vi "RTM - Remove Packet.vi"(8 "error in (no error)":errorcluster, 11 "Node Ptr":T1 format="%.0x") -> (0 "error out":errorcluster)   [LabVIEW 2019, in "UDP-Custom-Device System Explorer.lvlib"]
uses:
  UDP-Custom-Device System Explorer.lvlib
  <vilib>/NI VeriStand/Custom Device API/Custom Device Item Ref.ctl
  <vilib>/NI VeriStand/Custom Device Tools/Custom Device Utility Library/Custom Device Utility Library.lvlib
  <vilib>/NI VeriStand/Custom Device API/Custom Device API.lvlib
  Property Accessors/Shared Section Accessors.lvlib
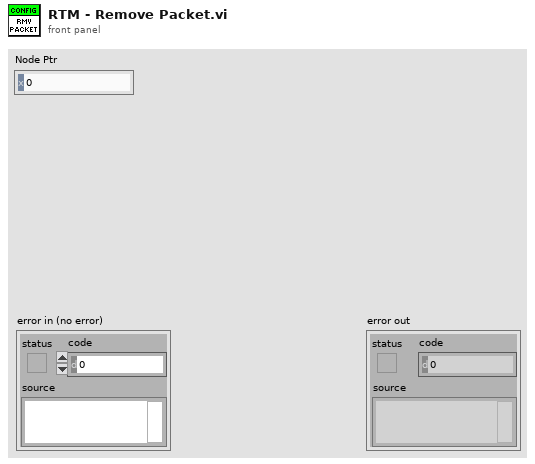
[diagram p1: front panel]
types:
  T1 = typedef "Custom Device API.lvlib/Custom Device Item Ref.ctl" = u64
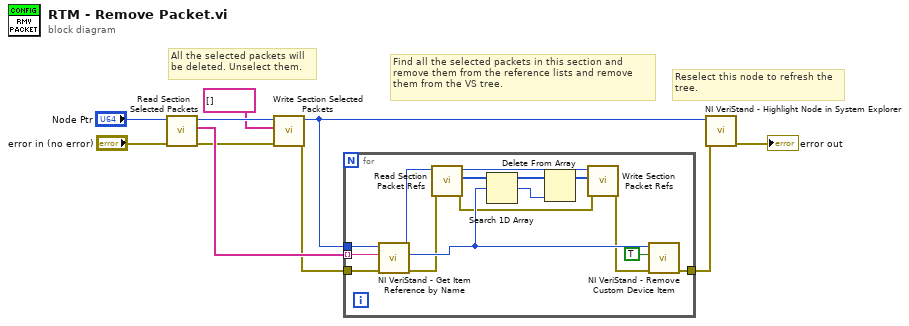
[diagram p0: block diagram]
diagram:
  # "All the selected packets will\nbe deleted. Unselect them."
  # "Reselect this node to refresh the\ntree."
  # "Find all the selected packets in this section and\nremove them from the reference lists and remove\nthem from the VS tree."
  n1 = call "Read Section Selected Packets.vi"("error in (no error)"="error in (no error)", "Node Ptr"="Node Ptr") -> ("error out"=w5:errorcluster, "Selected Packets"=w8:string[], "Node Ptr out"=w7:T1)  [unwired: 7 in]
  n2 = call "Write Section Selected Packets.vi"("error in (no error)"=w5, "Selected Packets"=string[] [] ("Value"), "Node Ptr"=w7) -> ("error out"=w4:errorcluster, "Node Ptr out"=w6:T1)  [unwired: 7 in]
  n3 = for {
    tunnel: w8 -> [w21] mode=indexing
    tunnel: w4 -> [w20]
    tunnel: [w24] -> w10
    tunnel: w6 -> [w22]
    n4 = call <vilib>:"NI VeriStand - Get Item Reference by Name.vi"("error in (no error)"=w20, "Item Name"=w21, "Parent Ref in"=w22) -> ("error out"=w13:errorcluster, "Item Ref"=w18:T1, "Parent Ref out"=w16:T1)  [unwired: 5 in, 1 out]
    n5 = call "Read Section Packet Refs.vi"("error in (no error)"=w13, "Node Ptr"=w16) -> ("error out"=w11:errorcluster, "Dependent Node Refs"=w15:T1[], "Node Ptr out"=w17:T1)  [unwired: 7 in]
    n6 = Search 1D Array(1D array=w15, element=w18) -> (index of element=w19:i32)  [unwired: 1 in]
    n7 = Delete From Array(array=w15, index=w19) -> (array with subset deleted=w14:T1[])  [unwired: 1 in, 1 out]
    n8 = call "Write Section Packet Refs.vi"("error in (no error)"=w11, "Dependent Node Refs"=w14, "Node Ptr"=w17) -> ("error out"=w12:errorcluster)  [unwired: 7 in, 1 out]
    n9 = call <vilib>:"NI VeriStand - Remove Custom Device Item.vi"("error in (no error)"=w12, "Force Delete (F)"=TRUE, "Item Ref in"=w18) -> ("error out"=w24:errorcluster)  [unwired: 7 in, 1 out]
  }
  n10 = call <vilib>:"NI VeriStand - Highlight Node in System Explorer.vi"("error in (no error)"=w10, "Item Ref in"=w6) -> ("error out"=→"error out":errorcluster)  [unwired: 8 in, 1 out]
